vi "Set Relation Definition.vi"(10 "Relation Definition":T1, 11 "Relation in":refnum<class "Relation.lvclass">) -> (3 "Relation out":refnum<class "Relation.lvclass">)   [LabVIEW 2020, in "Conditu2.lvlib" / "Columns.lvlib" / "Relation.lvclass"]
uses:
  Relation.lvclass
  Relation Info.ctl
  Relation Mapping.ctl
  Relation.lvclass/Relation.ctl
  Conditu2.lvlib
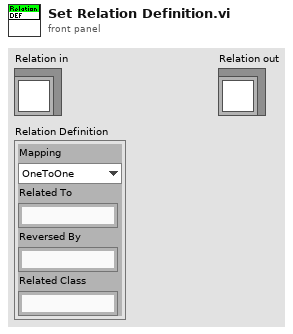
[diagram p1: front panel]
types:
  T1 = typedef "Conditu2.lvlib/Relation Info.ctl" = cluster{"Mapping":T2, "Related To":string, "Reversed By":string, "Related Class":string}
  T2 = typedef "Conditu2.lvlib/Relation Mapping.ctl" = enum16{"OneToOne", "OneToMany", "ManyToOne", "ManyToMany"}
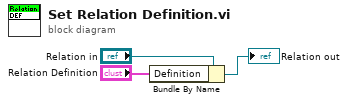
[diagram p0: block diagram]
diagram:
  n1 = Bundle By Name(cluster="Relation in", "Definition"="Relation Definition") -> (→"Relation out":refnum<class "Relation.lvclass">)
